vi "solar_msg UE Generate.vi"(4 "CMD_DATA (Array)":variant[](array[variant]), 6 "CMD (Array)":string[](array[string]), 7 "Priority? (F)":bool, 8 "error in (no error)":errorcluster, 9 "CMD_DATA (Last)":variant, 10 "CMD (Last)":string, 11 "UserEvent in":refnum<user-event>) -> (0 "error out":errorcluster, 3 "UserEvent":refnum<user-event>)   [LabVIEW 2018]
doc: "This generates a user event. The <b>CMD (Array)</b> is generated before the <b>CMD (Last)</b> is sent. <b>Priority?</b> generates a user event to the font."
uses:
  <vilib>/event_ctls.llb/usereventprio.ctl
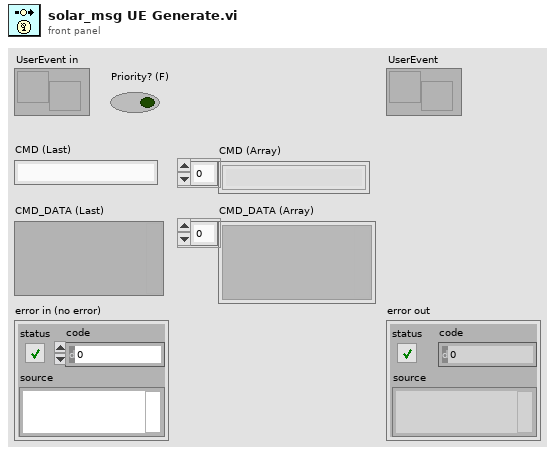
[diagram p1: front panel]
types:
  T1 = typedef "usereventprio.ctl" = enum32{"high priority", "normal priority"}
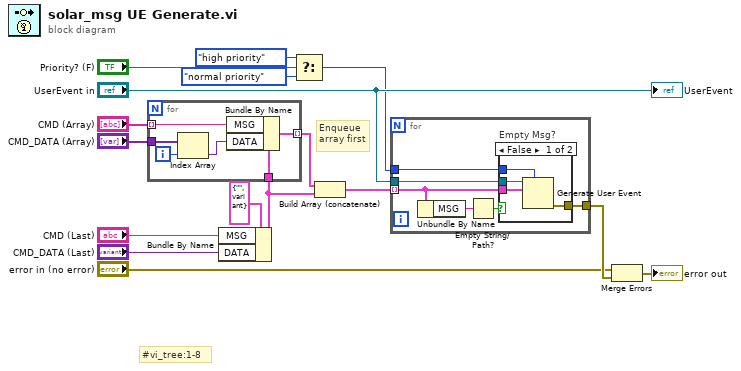
[diagram p0: block diagram]
diagram:
  # "#vi_tree:1-8"
  # "Enqueue\narray first"
  n1 = Bundle By Name(cluster=cluster{"MSG":string, "DATA":variant} {"MSG"="", "DATA"=variant} ("MSG"), "MSG"="CMD (Last)", "DATA"="CMD_DATA (Last)") -> (w7:cluster{"MSG":string, "DATA":variant})
  n2 = for {
    tunnel: "CMD (Array)" -> [w22] mode=indexing
    tunnel: "CMD_DATA (Array)" -> [w19]
    tunnel: w7 -> [w20]
    tunnel: [w21] -> w9 mode=indexing
    i -> [w18]
    n3 = Index Array(array=w19, index=w18) -> (element=w17:variant)
    n4 = Bundle By Name(cluster=w20, "MSG"=w22, "DATA"=w17) -> (w21:cluster{"MSG":string, "DATA":variant})
  }
  n5 = Select(t=usereventprio."high priority" ("priority (normal)"), s="Priority? (F)", f=usereventprio."normal priority" ("priority (normal)")) -> (s? t:f=w13:T1)
  n6 = Build Array (concatenate)(w9, w7) -> (w6:cluster{"MSG":string, "DATA":variant}[])
  n7 = for {
    tunnel: "UserEvent in" -> [w28]
    tunnel: [w27] -> w14
    tunnel: w13 -> [w26]
    tunnel: w6 -> [w25] mode=indexing
    n8 = Unbundle By Name(w25) -> ("MSG"=w24:string)
    n9 = Empty String/Path?(string/path=w24) -> (empty?=w23:bool)
    n10 = case "Empty Msg?" shown="False" w23 {
      tunnel: w28 -> [w32 _]
      tunnel: [w31 _] -> w27
      tunnel: w26 -> [w29 _]
      tunnel: w25 -> [w30 _]
      frame False {
        n11 = Generate User Event(priority (normal)=w29, user event=w32, event data cluster=w30) -> (error out=w31:errorcluster)  [unwired: 1 in, 1 out]
      }
      frame True {
      }
    }
  }
  n12 = Merge Errors("error in (no error)", w14) -> (→"error out":errorcluster)
  "UserEvent" <- "UserEvent in"
